vi "Add Regex Scrubber Unique.vi"   [LabVIEW 2020, in "Approval Tests.lvlib"]
doc: "Drops everything needed to scrub a particular regex with a counter that keeps track of unique values."
uses:
  Approval Tests.lvlib
  Options/Options.lvclass
  Regex Scrubber Count Unique/Regex Scrubber Count Unique.lvclass
  C:/Users/SAS/Desktop/ApprovalTests.LabVIEW/Source/Approval Tests/Scrubber/Scrubber.lvclass
  Regex Scrubber Count Unique/Regex Scrubber Count Unique.lvclass/Regex Scrubber Count Unique.ctl
  Regex Scrubber Count Unique/Write Regex.vi
  Regex Scrubber Count Unique/Write Prefix.vi
  Options/Write Add Scrubber.vi
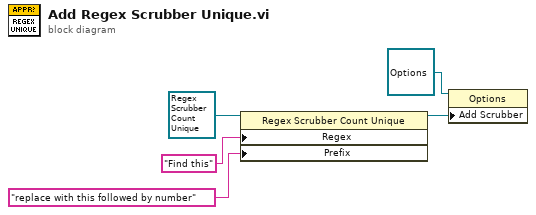
[diagram p0: block diagram]
diagram:
  n1 = property class="Regex Scrubber Count Unique"(reference=refnum<class "Regex Scrubber Count Unique.lvclass"> refnum ("Approval Tests.lvlib:Regex Scrubber Count Unique"), "Regex"="Find this", "Prefix"="replace with this followed by number" ("Replacement")) -> (reference out=w1:refnum<class "Regex Scrubber Count Unique.lvclass">)  [unwired: 1 in, 1 out]
  n2 = property class="Options"(reference=refnum<class "Options.lvclass"> refnum ("Approval Tests.lvlib:Options"), "Add Scrubber"=w1) -> ()  [unwired: 1 in, 2 out]
